vi "Find Pass or Fail.vi"(0 "Test Sequence Context":T1, 1 "Test Parameters":T3 {"Allowed Tolerance (%) FS" format="%#_4g"}, 2 "Sensor CoreData":T4, 3 "UUT Waveform":waveform(dbl), 4 "Reference Waveform":waveform(dbl), 5 "Setpoint Waveform":waveform(dbl), 7 "error in (no error)":errorcluster) -> (21 "New Processed Calibration Point":T7, 27 "error out":errorcluster)   [LabVIEW 2026, in "Processing_Engine.lvlib"]
uses:
  Processing_Engine.lvlib
  controls/Messaging Payloads/Processed Calibration Point.ctl
  controls/UI/Direction.ctl
  Test Status.ctl
  controls/Messaging Payloads/Sensor CoreData Cluster.ctl
  controls/UI/Units Enum.ctl
  controls/UI/Signal Enum.ctl
  Test Parameters Cluster.ctl
  controls/UI/Test Sequence Context.ctl
  <vilib>/Analysis/baseanly.llb/Mean (DBL).vi
  <vilib>/Analysis/NI_AALBase.lvlib
  Settings/Settings.lvlib
  Analysis/Analysis.lvlib
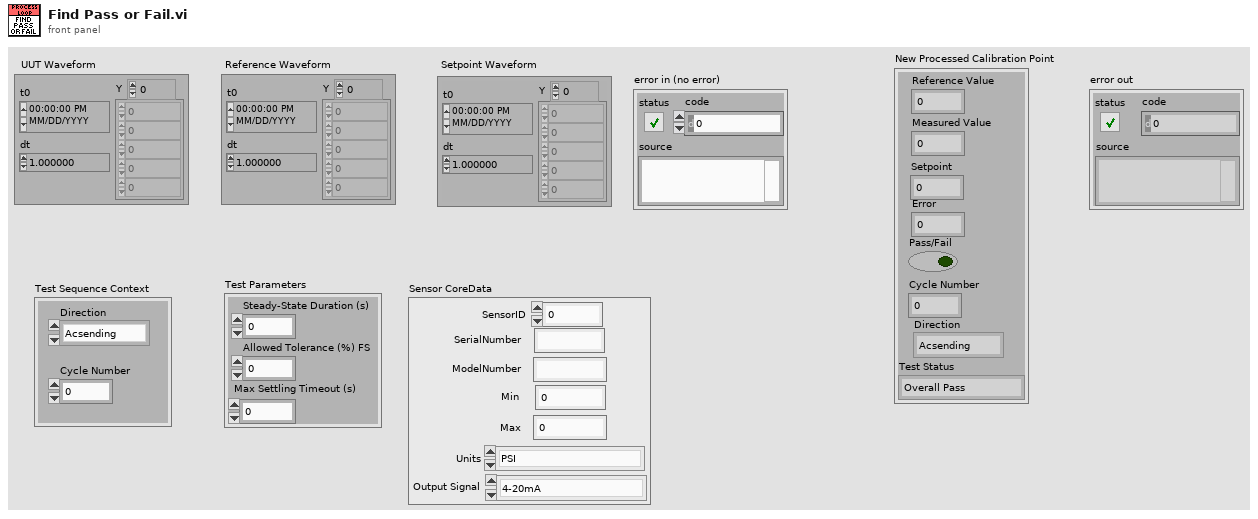
[diagram p1: front panel]
types:
  T1 = typedef "Settings.lvlib/Test Sequence Context.ctl" = cluster{"Direction":T2, "Cycle Number":i32}
  T2 = typedef "Settings.lvlib/Direction.ctl" = enum16{"Acsending", "Descending"}
  T3 = typedef "Settings.lvlib/Test Parameters Cluster.ctl" = cluster{"Steady-State Duration (s)":i32, "Allowed Tolerance (%) FS":dbl, "Max Settling Timeout (s)":i32}
  T4 = typedef "Settings.lvlib/Sensor CoreData Cluster.ctl" = cluster{"SerialNumber":string, "ModelNumber":string, "Min":dbl, "Max":dbl, "Units":T5, "Output Signal":T6, "SensorID":i32}
  T5 = typedef "Units Enum.ctl" = enum16{"PSI", "Deg C", "kPa", "GPM"}
  T6 = typedef "Signal Enum.ctl" = enum16{"4-20mA", "0-10V", "Thermocouple Type K"}
  T7 = typedef "Processed Calibration Point.ctl" = cluster{"Reference Value":dbl, "Measured Value":dbl, "Error":dbl, "Pass/Fail":bool, "Setpoint":dbl, "Cycle Number":i32, "Direction":T2, "Test Status":T8}
  T8 = typedef "Analysis.lvlib/Test Status.ctl" = enum16{"Overall Pass", "Overall Fail", "Test Running"}
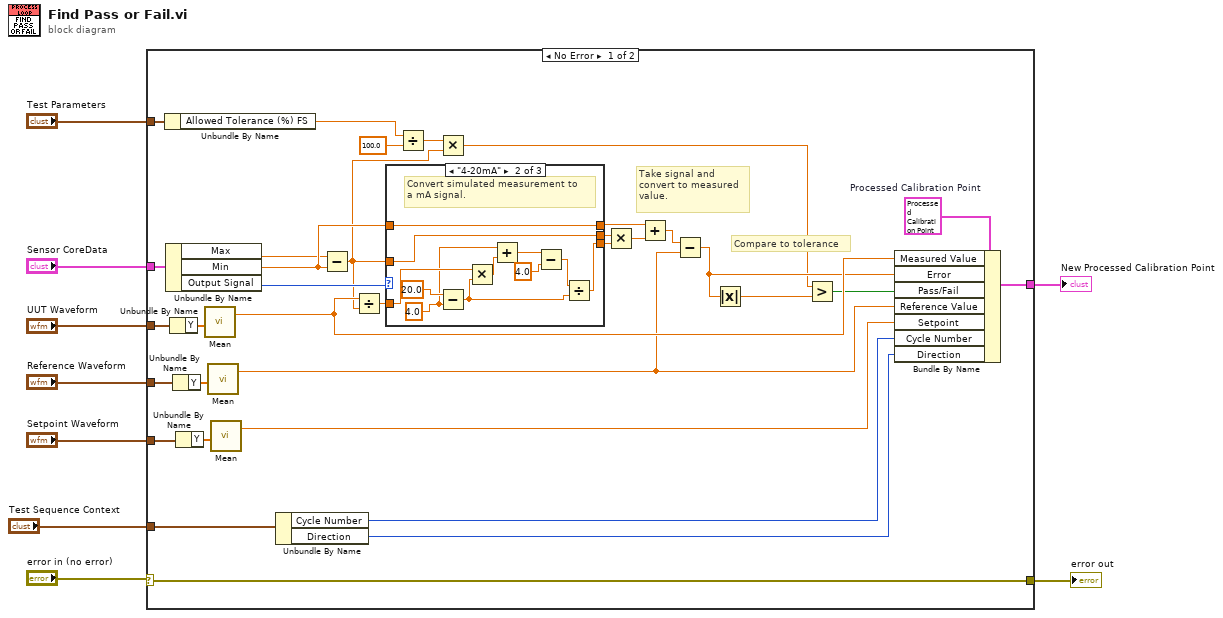
[diagram p0: block diagram]
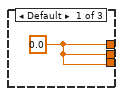
[diagram p2: hidden frame]
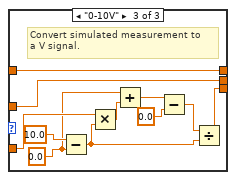
[diagram p3: hidden frame]
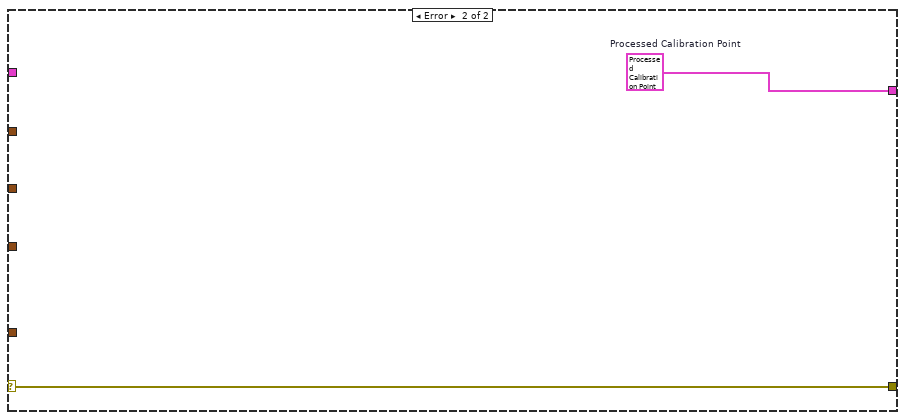
[diagram p4: hidden frame]
diagram:
  n1 = case shown="No Error" "error in (no error)" {
    selector: "error in (no error)" -> [w26 w68]
    tunnel: [w43 w67] -> w9
    tunnel: "Sensor CoreData" -> [w39 _]
    tunnel: "Test Parameters" -> [w28 _]
    tunnel: "UUT Waveform" -> [w27 _]
    tunnel: [w26 w68] -> w4
    tunnel: "Reference Waveform" -> [w24 _]
    tunnel: "Setpoint Waveform" -> [w19 _]
    tunnel: "Test Sequence Context" -> [w10 _]
    frame No Error {
      w40 = T7 {"Reference Value"=0.0, "Measured Value"=0.0, "Error"=0.0, "Pass/Fail"=FALSE, "Setpoint"=0.0, "Cycle Number"=0, "Direction"=enum."Acsending", "Test Status"=enum."Overall Pass"}  # Processed Calibration Point
      # "Compare to tolerance"
      # "Take signal and \nconvert to measured\nvalue."
      n2 = Unbundle By Name(w28) -> ("Allowed Tolerance (%) FS"=w16:dbl)
      n3 = Unbundle By Name(w39) -> ("Max"=w30:dbl, "Min"=w32:dbl, "Output Signal"=w31:T6)
      n4 = Unbundle By Name(w27) -> ("Y"=w38:dbl[])
      n5 = Unbundle By Name(w24) -> ("Y"=w25:dbl[])
      n6 = Unbundle By Name(w19) -> ("Y"=w21:dbl[])
      n7 = call-poly <vilib>:"Mean.vi"("X"=w38) -> ("mean"=w41:dbl)  [unwired: 1 out]
      n8 = call-poly <vilib>:"Mean.vi"("X"=w25) -> ("mean"=w22:dbl)  [unwired: 1 out]
      n9 = call-poly <vilib>:"Mean.vi"("X"=w21) -> ("mean"=w20:dbl)  [unwired: 1 out]
      n10 = Unbundle By Name(w10) -> ("Cycle Number"=w18:i32, "Direction"=w17:T2)
      n11 = Subtract(x=w30, y=w32) -> (x-y=w13:dbl)
      n12 = Divide(x=w41, y=w13) -> (x/y=w42:dbl)
      n13 = case shown="\"4-20mA\"" w31 {
        tunnel: w32 -> [_ w52 w63]
        tunnel: w13 -> [_ w50 w61]
        tunnel: [w44 w52 w63] -> w34
        tunnel: [w44 w51 w62] -> w35
        tunnel: [w44 w50 w61] -> w36
        tunnel: w42 -> [_ w49 w60]
        frame Default {
          w44 = 0.0 ("Min")
        }
        frame "4-20mA" {
          w46 = 4.0
          # "Convert simulated measurement to\na mA signal."
          n14 = Subtract(x=20.0, y=w46) -> (x-y=w48:dbl)
          n15 = Multiply(x=w49, y=w48) -> (x*y=w47:dbl)
          n16 = Add(x=w46, y=w47) -> (x+y=w45:dbl)
          n17 = Subtract(x=w45, y=4.0) -> (x-y=w53:dbl)
          n18 = Divide(x=w53, y=w48) -> (x/y=w51:dbl)
        }
        frame "0-10V" {
          w57 = 0.0
          # "Convert simulated measurement to\na V signal."
          n19 = Subtract(x=10.0, y=w57) -> (x-y=w59:dbl)
          n20 = Multiply(x=w60, y=w59) -> (x*y=w58:dbl)
          n21 = Add(x=w57, y=w58) -> (x+y=w56:dbl)
          n22 = Subtract(x=w56, y=0.0) -> (x-y=w64:dbl)
          n23 = Divide(x=w64, y=w59) -> (x/y=w62:dbl)
        }
      }
      n24 = Divide(x=w16, y=100.0) -> (x/y=w14:dbl)
      n25 = Multiply(x=w14, y=w13) -> (x*y=w12:dbl)
      n26 = Multiply(x=w36, y=w35) -> (x*y=w33:dbl)
      n27 = Add(x=w34, y=w33) -> (x+y=w23:dbl)
      n28 = Subtract(x=w23, y=w22) -> (x-y=w29:dbl)
      n29 = Absolute Value(x=w29) -> (abs(x)=w37:dbl)
      n30 = Greater?(x=w12, y=w37) -> (0:w11:bool)
      n31 = Bundle By Name(cluster=w40, "Measured Value"=w41, "Error"=w29, "Pass/Fail"=w11, "Reference Value"=w22, "Setpoint"=w20, "Cycle Number"=w18, "Direction"=w17) -> (w43:T7)
    }
    frame Error {
      w67 = T7 {"Reference Value"=0.0, "Measured Value"=0.0, "Error"=0.0, "Pass/Fail"=FALSE, "Setpoint"=0.0, "Cycle Number"=0, "Direction"=enum."Acsending", "Test Status"=enum."Overall Pass"}  # Processed Calibration Point
    }
  }
  "New Processed Calibration Point" <- w9
  "error out" <- w4
